vi "Pre-Build Action.vi"(10 "Variant":variant) -> (0 "error out":errorcluster)   [LabVIEW 2014]
uses:
  <vilib>/Utility/traverseref.llb/TRef TravTarget.ctl
  <vilib>/Utility/traverseref.llb/VI Scripting - Traverse.lvlib
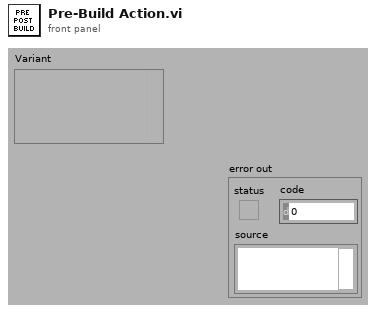
[diagram p1: front panel]
types:
  T1 = typedef "TRef TravTarget.ctl" = enum16{"FP", "BD", "Other"}
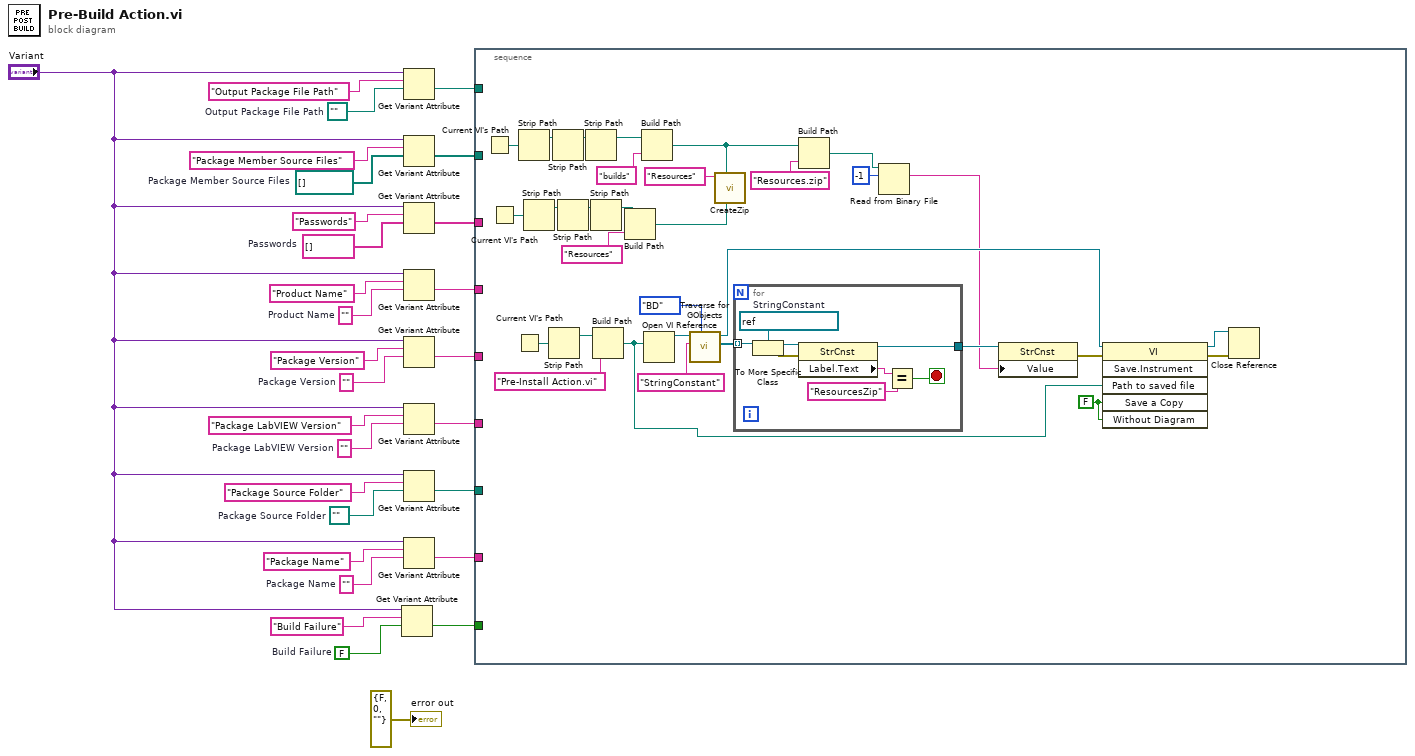
[diagram p0: block diagram]
diagram:
  w3 = FALSE  # Build Failure
  w13 = path ""  # Package Source Folder
  w14 = ""  # Package Name
  w17 = ""  # Package LabVIEW Version
  w19 = ""  # Package Version
  w21 = ""  # Product Name
  w24 = string[] []  # Passwords
  w26 = path[] []  # Package Member Source Files
  w28 = path ""  # Output Package File Path
  n1 = Get Variant Attribute(Variant="Variant", name="Build Failure", default value (empty Variant)=w3) -> (value=w1:bool)  [unwired: 1 in, 3 out]
  n2 = Get Variant Attribute(Variant="Variant", name="Output Package File Path", default value (empty Variant)=w28) -> (value=w12:path)  [unwired: 1 in, 3 out]
  n3 = Get Variant Attribute(Variant="Variant", name="Package Member Source Files", default value (empty Variant)=w26) -> (value=w11:path[])  [unwired: 1 in, 3 out]
  n4 = Get Variant Attribute(Variant="Variant", name="Passwords", default value (empty Variant)=w24) -> (value=w10:string[])  [unwired: 1 in, 3 out]
  n5 = Get Variant Attribute(Variant="Variant", name="Product Name", default value (empty Variant)=w21) -> (value=w9:string)  [unwired: 1 in, 3 out]
  n6 = Get Variant Attribute(Variant="Variant", name="Package Version", default value (empty Variant)=w19) -> (value=w8:string)  [unwired: 1 in, 3 out]
  n7 = Get Variant Attribute(Variant="Variant", name="Package LabVIEW Version", default value (empty Variant)=w17) -> (value=w7:string)  [unwired: 1 in, 3 out]
  n8 = Get Variant Attribute(Variant="Variant", name="Package Source Folder", default value (empty Variant)=w13) -> (value=w6:path)  [unwired: 1 in, 3 out]
  n9 = Get Variant Attribute(Variant="Variant", name="Package Name", default value (empty Variant)=w14) -> (value=w5:string)  [unwired: 1 in, 3 out]
  n10 = stacked-sequence {
    tunnel: w12 -> [_]
    tunnel: w11 -> [_]
    tunnel: w10 -> [_]
    tunnel: w9 -> [_]
    tunnel: w8 -> [_]
    tunnel: w7 -> [_]
    tunnel: w6 -> [_]
    tunnel: w5 -> [_]
    tunnel: w1 -> [_]
    frame #0 {
      w33 = FALSE ("Save a Copy")
      n11 = Current VI's Path() -> (path=w52:path)
      n12 = Current VI's Path() -> (path=w60:path)
      n13 = Current VI's Path() -> (path=w46:path)
      n14 = Strip Path(path=w52) -> (stripped path=w53:path)  [unwired: 1 out]
      n15 = Strip Path(path=w60) -> (stripped path=w59:path)  [unwired: 1 out]
      n16 = Strip Path(path=w46) -> (stripped path=w45:path)  [unwired: 1 out]
      n17 = Strip Path(path=w53) -> (stripped path=w54:path)  [unwired: 1 out]
      n18 = Strip Path(path=w59) -> (stripped path=w58:path)  [unwired: 1 out]
      n19 = Strip Path(path=w54) -> (stripped path=w51:path)  [unwired: 1 out]
      n20 = Strip Path(path=w58) -> (stripped path=w57:path)  [unwired: 1 out]
      n21 = Build Path(base path=w45, name or relative path="Pre-Install Action.vi") -> (appended path=w34:path)
      n22 = Build Path(base path=w57, name or relative path="Resources") -> (appended path=w47:path)
      n23 = Build Path(base path=w51, name or relative path="builds") -> (appended path=w49:path)
      n24 = Open VI Reference(vi path=w34) -> (vi reference=w43:refnum<vi>)  [unwired: 5 in, 1 out]
      n25 = call <vilib>:"Traverse for GObjects.vi"("Traverse Target"=TRef_TravTarget."BD", "Class Name"="StringConstant", "VI Refnum"=w43) -> ("References"=w41:refnum<vi>[], "dup VI Refnum"=w37:refnum<vi>)  [unwired: 5 in, 2 out]
      n26 = call "CreateZip.vi"("Source Dir"=w47, "Destination Directory"=w49, "ZIP File Name"="Resources") -> ()  [unwired: 9 in]
      n27 = for {
        tunnel: w41 -> [w68] mode=indexing
        tunnel: [w61] -> w39
        stop <- w62 stop-if-true
        w67 = refnum<vi> refnum  # StringConstant
        n28 = To More Specific Class(target class=w67, reference=w68) -> (specific class reference=w66:refnum<vi>, error out=w65:errorcluster)  [unwired: 1 in]
        n29 = property class="StrCnst"(reference=w66, error in=w65) -> (reference out=w61:refnum<vi>, "Label.Text"=w64:string)  [unwired: 1 out]
        n30 = Equal?(x=w64, y="ResourcesZip") -> (x = y?=w62:bool)
      }
      n31 = Build Path(base path=w49, name or relative path="Resources.zip" ("ZIP File Name")) -> (appended path=w32:path)
      n32 = Read from Binary File(10:-1 ("count (1)"), 11:w32) -> (2:w31:string)  [unwired: 4 in, 3 out]
      n33 = property class="StrCnst"(reference=w39, "Value"=w31) -> (error out=w38:errorcluster)  [unwired: 1 in, 1 out]
      n34 = invoke class="VI" method="Save.Instrument"(reference=w37, error in=w38, "Path to saved file"=w34, "Save a Copy"=w33, "Without Diagram"=w33) -> (reference out=w35:refnum<vi>, error out=w36:errorcluster)  [unwired: 1 in, 4 out]
      n35 = Close Reference(reference=w35, error in (no error)=w36) -> ()  [unwired: 1 out]
    }
  }
  "error out" <- errorcluster {"status"=FALSE, "code"=0, "source"=""} ("error out")
